vi "API_Call.vi"(0 "API Function Array":cluster{string, "VI Reference":refnum<vi>}[](array[cluster]), 1 "Argument List In":string[](array[string]), 2 "State":enum16{"Edit", "Start", "Run", "End", "Idle"}(ring), 3 "Elapsed Time (s)":dbl, 4 "Debug Mode":bool) -> (5 "Argument List Out":string[](array[string]), 6 "Status Out":string)   [LabVIEW 2011]
doc: "This VI implements functionality to call a polymorphic VI that implements the API function specification. To see an example of such an API function, examine Example.vi in the \"api\" directory. API_Call uses the argument list and the API Function array to locate the appropriate polymorphic reference stored in the API Function Array and execute it with the supplied state, elapsed time, and debug parameters."
panel:
  out "Error Out":errorcluster
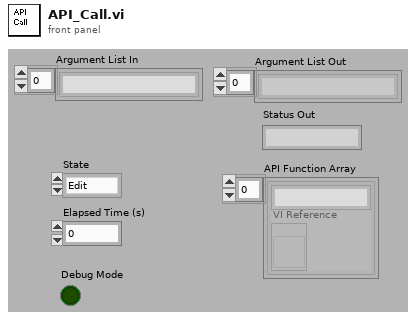
[diagram p1: front panel]
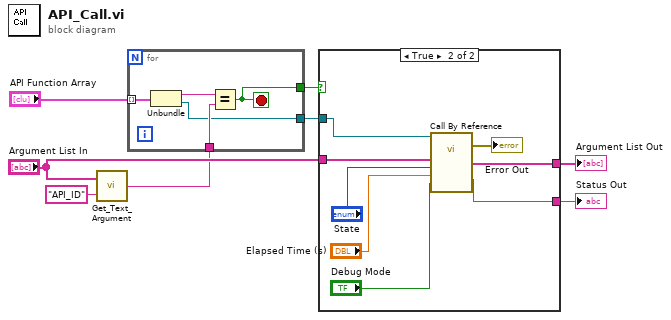
[diagram p0: block diagram]
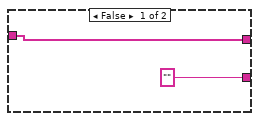
[diagram p2: hidden frame]
diagram:
  n1 = call "Get_Text_Argument.vi"("Argument"="API_ID", "Argument List"="Argument List In") -> ("Text"=w3:string)
  n2 = for {
    tunnel: "API Function Array" -> [w13] mode=indexing
    tunnel: w3 -> [w11]
    tunnel: [w10] -> w2
    tunnel: [w9] -> w1
    stop <- w10 stop-if-true
    n3 = Unbundle(w13) -> (w12:string, "VI Reference"=w9:refnum<vi>)
    n4 = Equal?(x=w12, y=w11) -> (x = y?=w10:bool)
  }
  n5 = case shown="True" w2 {
    tunnel: "Argument List In" -> [w14 w20]
    tunnel: [w14 w19] -> w5
    tunnel: ["" ("Status Out") w18] -> w4
    tunnel: w1 -> [_ w17]
    frame False {
    }
    frame True {
      n6 = call-by-ref "?"(reference=w17, "Debug Mode"="Debug Mode", "Elapsed Time (s)"="Elapsed Time (s)", "State"="State", "Argument List In"=w20) -> (error out=→"Error Out":errorcluster, "Status Out"=w18:string, "Argument List Out"=w19:string[])  [unwired: 1 in, 1 out]
    }
  }
  "Argument List Out" <- w5
  "Status Out" <- w4
